vi "ConvertArrayToWaveform.vi"(6 "Scaling [dB]":dbl, 8 "Remove DC":bool, 9 "Input Array":dbl[](array[numeric]), 10 "Voltage Conversion Factor [V]":dbl, 11 "Sample Rate [Hz]":u32) -> (3 "Output Waveform":waveform(dbl))   [LabVIEW 2020]
uses:
  <vilib>/Analysis/NI_AALPro.lvlib
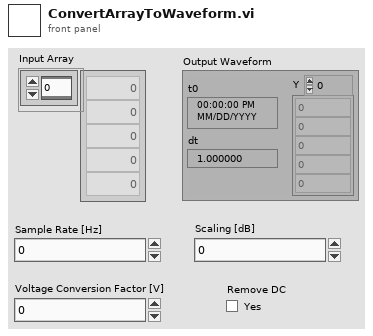
[diagram p1: front panel]
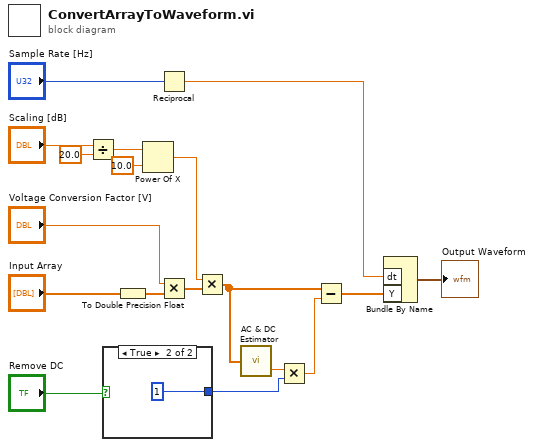
[diagram p0: block diagram]
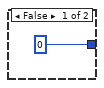
[diagram p2: hidden frame]
diagram:
  n1 = Divide(x="Scaling [dB]", y=20.0) -> (x/y=w2:dbl)
  n2 = case shown="True" "Remove DC" {
    tunnel: [0 1] -> w8
    frame False {
    }
    frame True {
    }
  }
  n3 = To Double Precision Float(number="Input Array") -> (double precision float=w14:dbl[])
  n4 = Power Of X(1:10.0 ("x"), 2:w2) -> (0:w3:dbl)
  n5 = Reciprocal(x="Sample Rate [Hz]") -> (1/x=w13:dbl)
  n6 = Multiply(x="Voltage Conversion Factor [V]", y=w14) -> (x*y=w7:dbl[])
  n7 = Multiply(x=w3, y=w7) -> (x*y=w6:dbl[])
  n8 = call <vilib>:"AC & DC Estimator.vi"("Signal (V)"=w6) -> ("DC estimate (V)"=w10:dbl)  [unwired: 1 out]
  n9 = Multiply(x=w10, y=w8) -> (x*y=w9:dbl)
  n10 = Subtract(x=w6, y=w9) -> (x-y=w12:dbl[])
  n11 = Bundle By Name("dt"=w13, "Y"=w12) -> (→"Output Waveform":waveform(dbl))  [unwired: 1 in]
